vi "SetParameter_popup.vi"(0 "Input Line Command":string, 3 "error in (no error)":errorcluster, 4 "Control Name":string, 5 "Control Type":string(combo)="String", 7 "Value":string) -> (8 "error out":errorcluster, 9 "Cancel":bool, 10 "Output Line Command":string)   [LabVIEW 2025]
uses:
  <vilib>/Utility/error.llb/Trim Whitespace One-Sided.vi
panel:
  in  "Remote computer IP:Port":string
  in  "platform":u16(ring) items=["Mac", "PC"]
  in  "Target VI":string
  in  "Cancel button":bool
  in  "OK Button":bool
  # "(empty: local host)"
  # "Boolean, 0: False, 1: True"
  # "For the remote connection*\nNavigate to VI server settings of the host (remote)\n computer. (Menu: Tools-> Options -> VI server) \n\n(1) Protocols: TCP/IP enabled. Verifiy the port #.\n(2) Machine Access: add this computer's IP in the list.\n\n* Assuming the firewall setting (requires administrator previleage) \nwas set to allow the LabView connection."
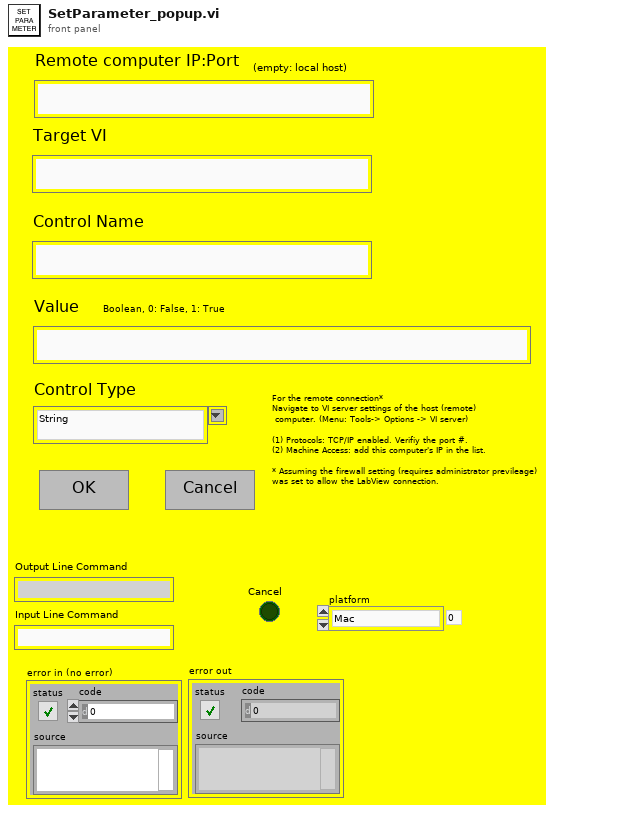
[diagram p1: front panel]
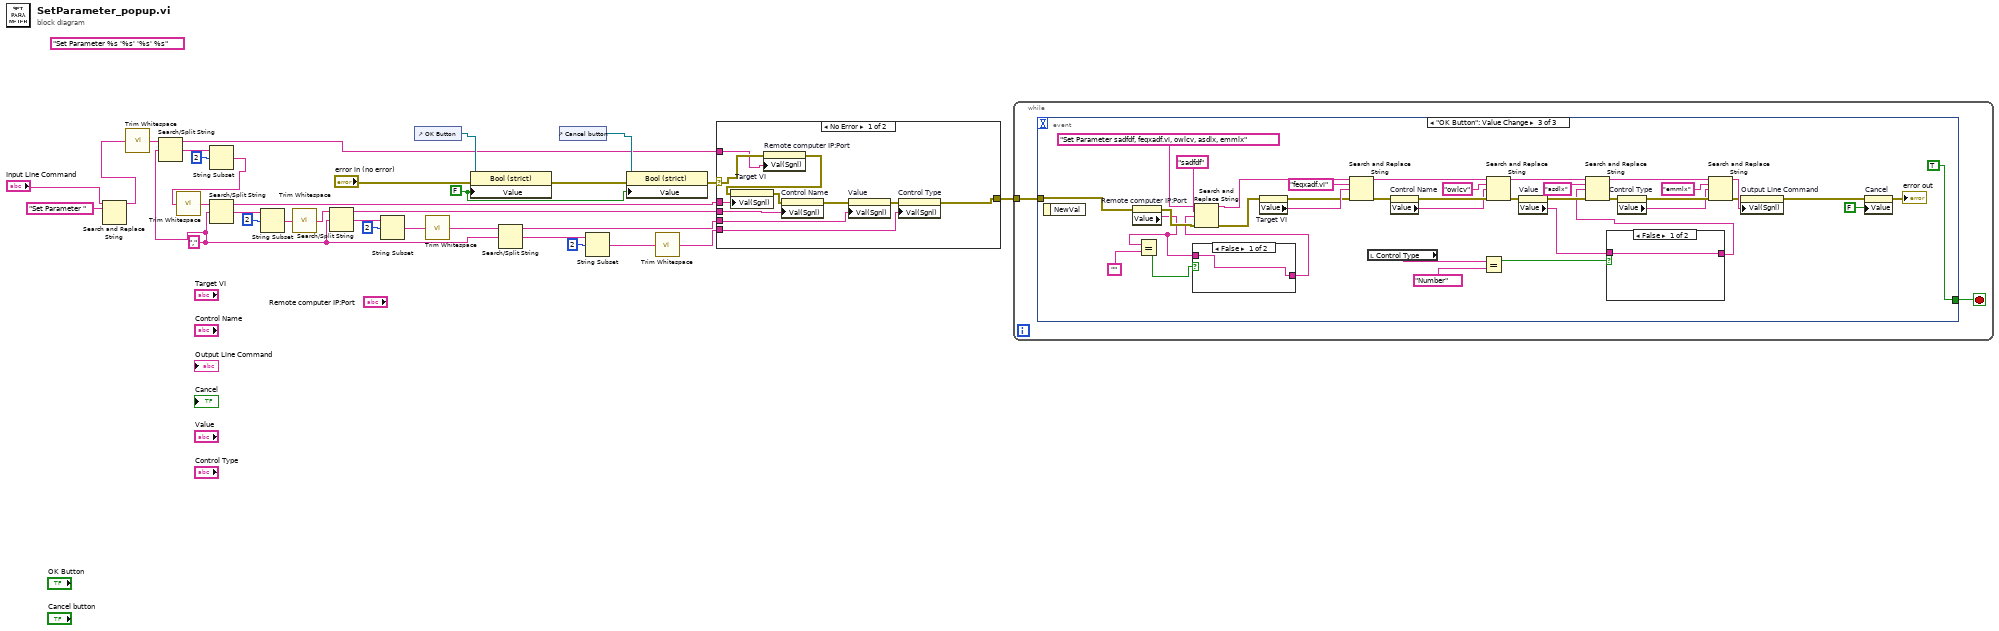
[diagram p0: block diagram]
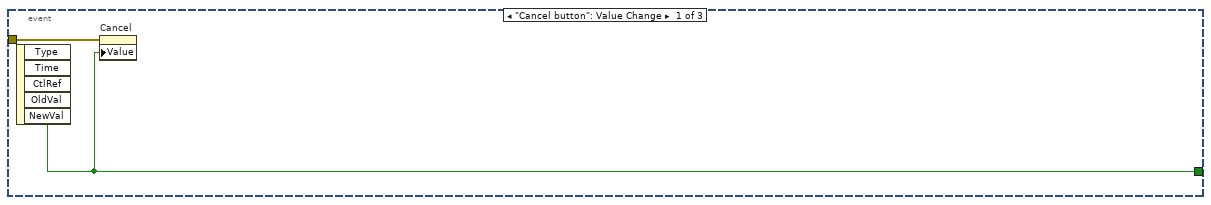
[diagram p2: hidden frame]
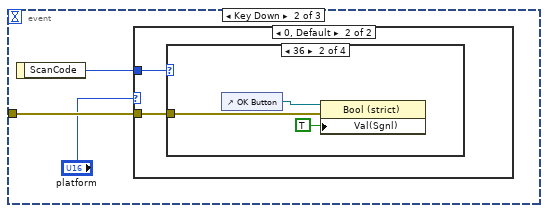
[diagram p3: hidden frame]
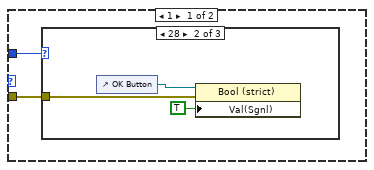
[diagram p4: hidden frame]
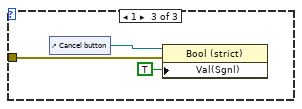
[diagram p6: hidden frame]
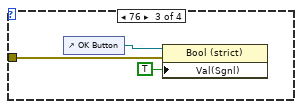
[diagram p8: hidden frame]
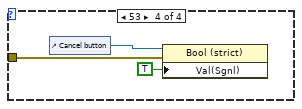
[diagram p9: hidden frame]
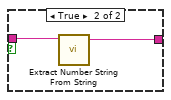
[diagram p10: hidden frame]
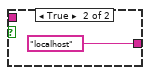
[diagram p11: hidden frame]
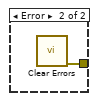
[diagram p12: hidden frame]
diagram:
  w3 = "," ("search string/char (-)")
  (unwired) "Set Parameter %s '%s' '%s' %s" ("format string")
  w32 = FALSE
  n1 = Search and Replace String(input string="Input Line Command", search string="Set Parameter ") -> (result string=w4:string)  [unwired: 6 in, 3 out]
  n2 = call <vilib>:"Trim Whitespace.vi"("string"=w4) -> ("trimmed string"=w7:string)  [unwired: 1 in]
  n3 = Search/Split String(string=w7, search string/char (-)=w3) -> (substring before match=w1:string, match + rest of string=w5:string)  [unwired: 1 in, 1 out]
  n4 = String Subset(string=w5, offset (0)=2) -> (substring=w2:string)  [unwired: 1 in]
  n5 = call <vilib>:"Trim Whitespace.vi"("string"=w2) -> ("trimmed string"=w23:string)  [unwired: 1 in]
  n6 = Search/Split String(string=w23, search string/char (-)=w3) -> (substring before match=w12:string, match + rest of string=w21:string)  [unwired: 1 in, 1 out]
  n7 = String Subset(string=w21, offset (0)=2) -> (substring=w20:string)  [unwired: 1 in]
  n8 = call <vilib>:"Trim Whitespace.vi"("string"=w20) -> ("trimmed string"=w25:string)  [unwired: 1 in]
  n9 = Search/Split String(string=w25, search string/char (-)=w3) -> (substring before match=w11:string, match + rest of string=w18:string)  [unwired: 1 in, 1 out]
  n10 = String Subset(string=w18, offset (0)=2) -> (substring=w17:string)  [unwired: 1 in]
  n11 = control-ref of="OK Button"() -> (w31:refnum<vi>)
  n12 = call <vilib>:"Trim Whitespace.vi"("string"=w17) -> ("trimmed string"=w24:string)  [unwired: 1 in]
  n13 = property on="Property Node" class="Bool (strict)"(reference=w31, error in="error in (no error)", "Value"=w32) -> (error out=w28:errorcluster)  [unwired: 1 out]
  n14 = Search/Split String(string=w24, search string/char (-)=w3) -> (substring before match=w10:string, match + rest of string=w15:string)  [unwired: 1 in, 1 out]
  n15 = control-ref of="Cancel button"() -> (w30:refnum<vi>)
  n16 = String Subset(string=w15, offset (0)=2) -> (substring=w14:string)  [unwired: 1 in]
  n17 = property on="Property Node" class="Bool (strict)"(reference=w30, error in=w28, "Value"=w32) -> (error out=w8:errorcluster)  [unwired: 1 out]
  n18 = call <vilib>:"Trim Whitespace.vi"("string"=w14) -> ("trimmed string"=w9:string)  [unwired: 1 in]
  n19 = case shown="No Error" w8 {
    selector: w8 -> [w35 _]
    tunnel: [w42 w44] -> w27
    tunnel: w12 -> [w39 _]
    tunnel: w11 -> [w38 _]
    tunnel: w10 -> [w37 _]
    tunnel: w9 -> [w36 _]
    tunnel: w1 -> [w33 _]
    frame No Error {
      n20 = property on="Remote computer IP:Port" class="Str"(error in=w35, "Val(Sgnl)"=w33) -> (error out=w34:errorcluster)  [unwired: 1 in, 1 out]
      n21 = property on="Target VI" class="Str"(error in=w34, "Val(Sgnl)"=w39) -> (error out=w40:errorcluster)  [unwired: 1 in, 1 out]
      n22 = property on="Control Name" class="Str"(error in=w40, "Val(Sgnl)"=w38) -> (error out=w41:errorcluster)  [unwired: 1 in, 1 out]
      n23 = property on="Value" class="Str"(error in=w41, "Val(Sgnl)"=w37) -> (error out=w43:errorcluster)  [unwired: 1 in, 1 out]
      n24 = property on="Control Type" class="CmbBox"(error in=w43, "Val(Sgnl)"=w36) -> (error out=w42:errorcluster)  [unwired: 1 in, 1 out]
    }
    frame Error {
      n25 = call <vilib>:"Clear Errors.vi"() -> ("error out"=w44:errorcluster)  [unwired: 6 in, 1 out]
    }
  }
  n26 = while {
    tunnel: w27 -> [w46]
    stop <- w45 stop-if-true
    n27 = event shown="[2] \"OK Button\": Value Change" {
      selector: _ -> [_ _ _]
      dyn-events: _ -> [_ _ _]
      timeout: _ -> [_ _ _]
      tunnel: w46 -> [w48 w50 w83]
      tunnel: [w47 _ TRUE] -> w45
      event "Cancel button": Value Change {
        n28 = event-data() -> ("NewVal"=w47:bool)  [unwired: 1 in, 4 out]
        n29 = property on="Cancel" class="Bool (strict)"(error in=w48, "Value"=w47) -> ()  [unwired: 1 in, 2 out]
      }
      event Key Down {
        n30 = event-data() -> ("ScanCode"=w51:i16)  [unwired: 1 in]
        n31 = case shown="0, Default" "platform" {
          tunnel: w51 -> [w53 w61]
          tunnel: w50 -> [w52 w60]
          frame 1 {
            n32 = case shown="28" w53 {
              tunnel: w52 -> [_ w56 w58]
              frame Default {
              }
              frame 28 {
                n33 = control-ref of="OK Button"() -> (w54:refnum<vi>)
                n34 = property on="Property Node" class="Bool (strict)"(reference=w54, error in=w56, "Val(Sgnl)"=TRUE ("Value (Signaling)")) -> ()  [unwired: 2 out]
              }
              frame 1 {
                n35 = control-ref of="Cancel button"() -> (w57:refnum<vi>)
                n36 = property on="Property Node" class="Bool (strict)"(reference=w57, error in=w58, "Val(Sgnl)"=TRUE ("Value (Signaling)")) -> ()  [unwired: 2 out]
              }
            }
          }
          frame 0, Default {
            n37 = case shown="36" w61 {
              tunnel: w60 -> [_ w64 w67 w69]
              frame Default {
              }
              frame 36 {
                n38 = control-ref of="OK Button"() -> (w62:refnum<vi>)
                n39 = property on="Property Node" class="Bool (strict)"(reference=w62, error in=w64, "Val(Sgnl)"=TRUE ("Value (Signaling)")) -> ()  [unwired: 2 out]
              }
              frame 76 {
                n40 = control-ref of="OK Button"() -> (w65:refnum<vi>)
                n41 = property on="Property Node" class="Bool (strict)"(reference=w65, error in=w67, "Val(Sgnl)"=TRUE ("Value (Signaling)")) -> ()  [unwired: 2 out]
              }
              frame 53 {
                n42 = control-ref of="Cancel button"() -> (w68:refnum<vi>)
                n43 = property on="Property Node" class="Bool (strict)"(reference=w68, error in=w69, "Val(Sgnl)"=TRUE ("Value (Signaling)")) -> ()  [unwired: 2 out]
              }
            }
          }
        }
      }
      event "OK Button": Value Change {
        n44 = event-data() -> ()  [unwired: 1 in, 1 out]
        n45 = property on="Remote computer IP:Port" class="Str"(error in=w83) -> (error out=w79:errorcluster, "Value"=w76:string)  [unwired: 1 in, 1 out]
        n46 = Equal?(x=w76, y="") -> (x = y?=w84:bool)
        n47 = case shown="False" w84 {
          tunnel: [w112 "localhost" ("search string")] -> w77
          tunnel: w76 -> [w112 _]
          frame False {
          }
          frame True {
          }
        }
        n48 = Search and Replace String(input string="Set Parameter sadfdf, feqxadf.vi, owlcv, asdlx, emmlx" ("format string"), search string="sadfdf", replace string=w77, error in=w79) -> (result string=w81:string, error out=w78:errorcluster)  [unwired: 4 in, 2 out]
        n49 = property on="Target VI" class="Str"(error in=w78) -> (error out=w87:errorcluster, "Value"=w88:string)  [unwired: 1 in, 1 out]
        n50 = Search and Replace String(input string=w81, search string="feqxadf.vi", replace string=w88, error in=w87) -> (result string=w90:string, error out=w86:errorcluster)  [unwired: 4 in, 2 out]
        n51 = local read "Control Type"() -> (w72:string)
        n52 = property on="Control Name" class="Str"(error in=w86) -> (error out=w101:errorcluster, "Value"=w100:string)  [unwired: 1 in, 1 out]
        n53 = Equal?(x=w72, y="Number" ("Control Type")) -> (x = y?=w71:bool)
        n54 = Search and Replace String(input string=w90, search string="owlcv", replace string=w100, error in=w101) -> (result string=w106:string, error out=w99:errorcluster)  [unwired: 4 in, 2 out]
        n55 = property on="Value" class="Str"(error in=w99) -> (error out=w98:errorcluster, "Value"=w75:string)  [unwired: 1 in, 1 out]
        n56 = case shown="False" w71 {
          tunnel: w75 -> [w109 w111]
          tunnel: [w109 w110] -> w74
          frame False {
          }
          frame True {
            n57 = call "Extract Number String From String.vi"("string"=w111) -> ("number string out"=w110:string)  [unwired: 5 in, 2 out]
          }
        }
        n58 = Search and Replace String(input string=w106, search string="asdlx", replace string=w74, error in=w98) -> (result string=w97:string, error out=w95:errorcluster)  [unwired: 4 in, 2 out]
        n59 = property on="Control Type" class="CmbBox"(error in=w95) -> (error out=w94:errorcluster, "Value"=w93:string)  [unwired: 1 in, 1 out]
        n60 = Search and Replace String(input string=w97, search string="emmlx", replace string=w93, error in=w94) -> (result string=w96:string, error out=w91:errorcluster)  [unwired: 4 in, 2 out]
        n61 = property on="Output Line Command" class="Str"(error in=w91, "Val(Sgnl)"=w96) -> (error out=w104:errorcluster)  [unwired: 1 in, 1 out]
        n62 = property on="Cancel" class="Bool (strict)"(error in=w104, "Value"=FALSE ("Cancel")) -> (error out=→"error out":errorcluster)  [unwired: 1 in, 1 out]
      }
    }
  }
